vi "CheckUnifiedActor.vi"(11 "Unified Actor":refnum<class "Actor.lvclass">) -> (3 "Error":errorcluster)   [LabVIEW 2020, in "jettl.lvlib"]
uses:
  jettl.lvlib
  Lifetime.ctl
  Actor/Actor.lvclass
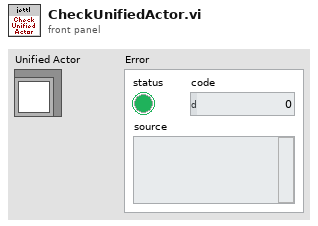
[diagram p1: front panel]
types:
  T1 = typedef "jettl.lvlib/Lifetime.ctl" = enum16{"Init", "Spawn", "Setup", "TeardownBeforeRunning", "Running", "StopCalled", "StoppingWithComponents", "StoppingNoComponents", "TeardownAfterRunning", "Stopped"}
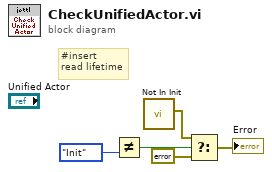
[diagram p0: block diagram]
diagram:
  # "#insert\nread lifetime"
  n1 = Not Equal?(y=Lifetime."Init") -> (x=w1:T1, x != y?=w4:bool)
  n2 = call "Not In Init.vi"() -> ("Error"=w7:errorcluster)  [unwired: 11 in]
  n3 = Select(t=w7, s=w4, f=errorcluster {"status"=FALSE, "code"=0, "source"=""}) -> (s? t:f=→"Error":errorcluster)
